vi "NamedRegAndResolve.vi"() -> ()   [LabVIEW 2024, in "Module Container.lvlib"]
uses:
  Module Container.lvlib
  ModuleCore/RQMHModule.lvclass
  ModuleTemplates/NewTemplateModule/NewTemplate.lvclass
panel:
  out "Shouldn't Error":errorcluster
  out "Should Error":errorcluster
  in  "stop":bool
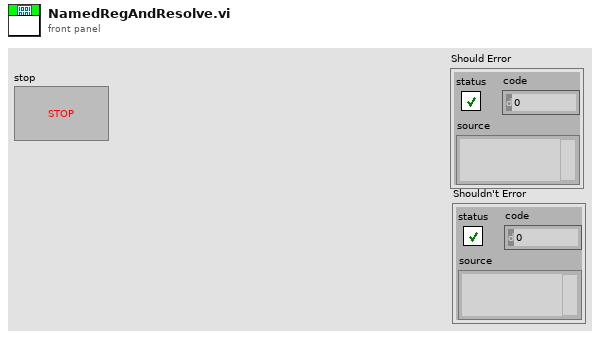
[diagram p1: front panel]
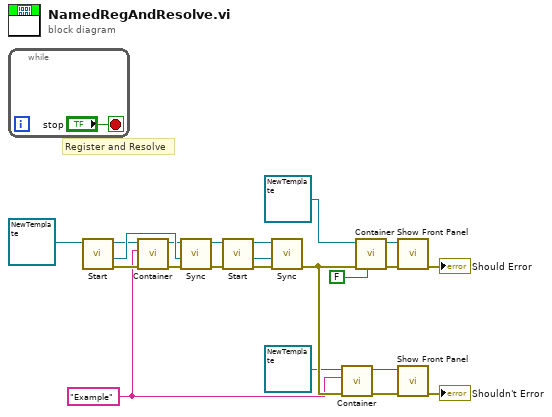
[diagram p0: block diagram]
diagram:
  w5 = "Example" ("Specific")
  # "Register and Resolve"
  n1 = while {
    stop <- "stop" stop-if-true
  }
  n2 = call "Start.vi"("JQMHCore in"=refnum<class "NewTemplate.lvclass"> refnum ("Template")) -> ("error out"=w14:errorcluster, "StartupHandshake out"=w22:refnum<class "RQMHStartup.lvclass">, "JQMHCore out"=w17:refnum<class "NewTemplate.lvclass">)  [unwired: 8 in]
  n3 = call "Container.vi"("error in (no error)"=w14, "Specific"=w5, "Module Type"=w17) -> ("error out"=w13:errorcluster, "Module Instance"=w16:refnum<class "NewTemplate.lvclass">)  [unwired: 6 in, 1 out]
  n4 = call "Sync.vi"("error in (no error)"=w13, "StartupHandshake out"=w22, "JQMHCore in"=w16) -> ("error out"=w4:errorcluster, "JQMHCore out"=w20:refnum<class "NewTemplate.lvclass">)  [unwired: 7 in]
  n5 = call "Start.vi"("error in (no error)"=w4, "JQMHCore in"=w20) -> ("error out"=w21:errorcluster, "StartupHandshake out"=w18:refnum<class "RQMHStartup.lvclass">, "JQMHCore out"=w19:refnum<class "NewTemplate.lvclass">)  [unwired: 7 in]
  n6 = call "Sync.vi"("error in (no error)"=w21, "StartupHandshake out"=w18, "JQMHCore in"=w19) -> ("error out"=w9:errorcluster)  [unwired: 7 in, 1 out]
  n7 = call "Container.vi"("error in (no error)"=w9, "Specific"=w5, "Module Type"=refnum<class "NewTemplate.lvclass"> refnum ("Template")) -> ("error out"=w8:errorcluster, "Module Instance"=w10:refnum<class "NewTemplate.lvclass">)  [unwired: 6 in, 1 out]
  n8 = call "Container.vi"("Start if not running? (T)"=FALSE, "error in (no error)"=w9, "Module Type"=refnum<class "NewTemplate.lvclass"> refnum ("Template")) -> ("error out"=w7:errorcluster, "Module Instance"=w15:refnum<class "NewTemplate.lvclass">)  [unwired: 6 in, 1 out]
  n9 = call "Show Front Panel.vi"("error in (no error)"=w7, "JQMHCore in"=w15) -> ("error out"=→"Should Error":errorcluster)  [unwired: 8 in, 1 out]
  n10 = call "Show Front Panel.vi"("error in (no error)"=w8, "JQMHCore in"=w10) -> ("error out"=→"Shouldn't Error":errorcluster)  [unwired: 8 in, 1 out]
